vi "libssh2_channel_request_pty_size_ex.vi"(4 "height_px":i32, 6 "width_px":i32, 8 "error in (no error)":errorcluster, 9 "height":i32=24, 10 "width":i32=80, 11 "channel":T1) -> (0 "error out":errorcluster)   [LabVIEW 2017, in "libssh2.lvlib"]
doc: "Change the size of a pseudo-terminal on a channel."
uses:
  libssh2.lvlib
  Channel Refnum.ctl
  Acquire Session.vi
  Release Session.vi
  Not A Channel.vi
  <vilib>/Utility/error.llb/Error Cluster From Error Code.vi
  Global Settings.vi
  Read Channel Refnum.vi
  Read Session Refnum.vi
  <vilib>/Utility/semaphor.llb/Acquire Semaphore.vi
  <vilib>/Utility/semaphor.llb/Release Semaphore.vi
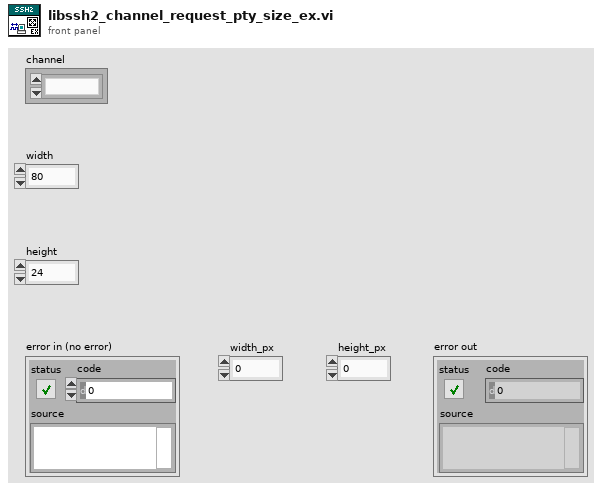
[diagram p1: front panel]
types:
  T1 = typedef "libssh2.lvlib/Channel Refnum.ctl" = refnum<k1>
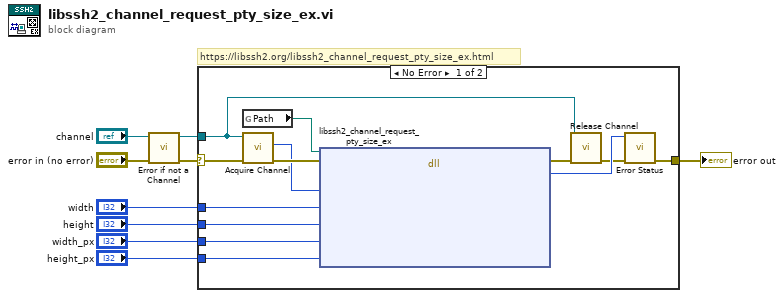
[diagram p0: block diagram]
diagram:
  # "https://libssh2.org/libssh2_channel_request_pty_size_ex.html"
  n1 = call "Error if not a Channel.vi"("error in (no error)"="error in (no error)", "channel"="channel") -> ("error out"=w7:errorcluster, "channel out"=w5:T1)  [unwired: 8 in]
  n2 = case shown="No Error" w7 {
    selector: w7 -> [w22 w23]
    tunnel: [w21 w23] -> w9
    tunnel: w5 -> [w10 _]
    tunnel: "width" -> [w15 _]
    tunnel: "height" -> [w14 _]
    tunnel: "width_px" -> [w13 _]
    tunnel: "height_px" -> [w12 _]
    frame No Error {
      n3 = global read "Global Settings.vi" "Path"() -> (w17:path)
      n4 = call "Acquire Channel.vi"("error in (no error)"=w22, "channel"=w10) -> ("error out"=w19:errorcluster, "LIBSSH2_CHANNEL*"=w18:u64)  [unwired: 8 in]
      n5 = dll-call lib="?" fn="libssh2_channel_request_pty_size_ex"(path in=w17, error in=w19, "channel"=w18, "width"=w15, "height"=w14, "width_px"=w13, "height_px"=w12) -> (error out=w20:errorcluster, "return value"=w16:i32)  [unwired: 6 in, 1 out]
      n6 = call "Release Channel.vi"("error in (no error)"=w20, "channel"=w10) -> ("error out"=w11:errorcluster)  [unwired: 9 in]
      n7 = call "Error Status.vi"("error in (no error)"=w11, "return value"=w16) -> ("error out"=w21:errorcluster)  [unwired: 8 in, 1 out]
    }
    frame Error {
    }
  }
  "error out" <- w9
